vi "CreateLib.vi"(0 "LibWriter":refnum<class "LibWriter.lvclass">, 1 "ProjectTreePosition(String or Project Item Ref)":variant, 2 "CreateLibData":T1, 5 "error in (no error)":errorcluster, 6 "KeepLvLibRefOpen(False)":bool, 7 "HeaderToApply (take from VIRef or /use 2D-8bit header, Ignored if not wired)":variant) -> (14 "LibWriter":refnum<class "LibWriter.lvclass">, 15 "LVLibLibraryRefnum":refnum<vi>, 16 "TemplateVersionUsed":string, 19 "error out":errorcluster)   [LabVIEW 2014, in "LibWriter.lvclass"]
uses:
  <resource>/Framework/Providers/Open_GDS/ClassProviders/LibProvider_BaseClassInterface/LibWriter_class/ClassWriter_class/LibWriter.lvclass
  <resource>/Framework/Providers/Open_GDS/ClassProviders/LibProvider_BaseClassInterface/LibWriter_class/CreateLibData.vi
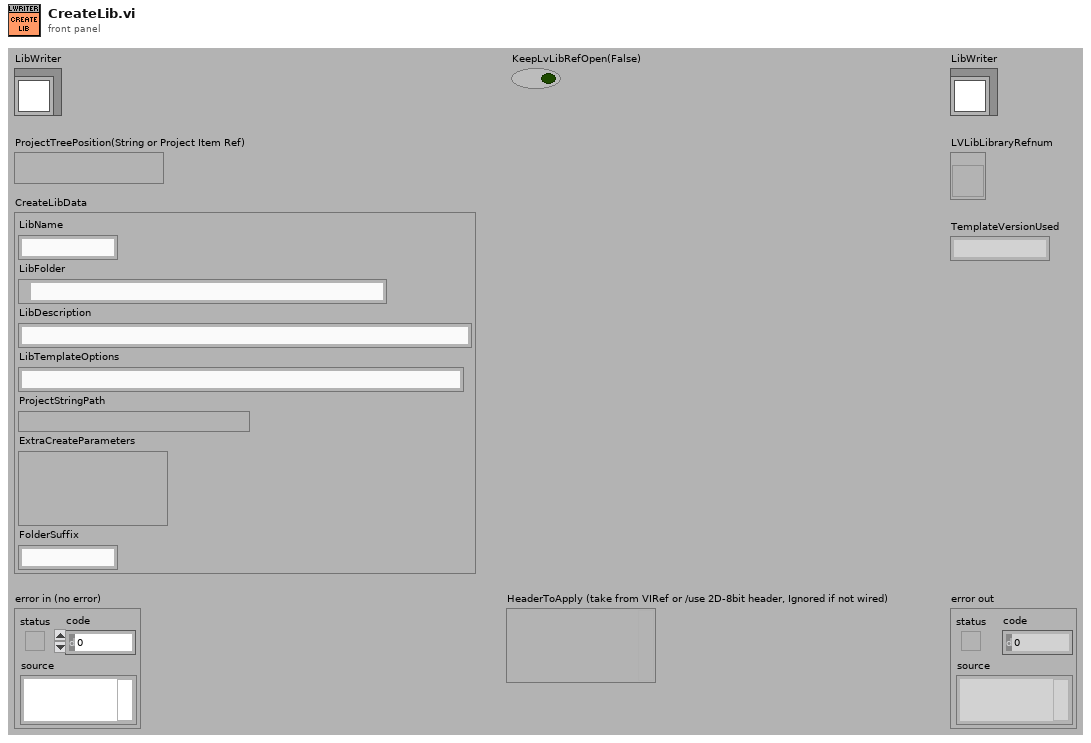
[diagram p1: front panel]
types:
  T1 = typedef "LibWriter.lvclass/CreateLibData.vi" = cluster{"LibName":string, "LibFolder":path, "LibDescription":string, "LibTemplateOptions":string, "ProjectStringPath":variant, "ExtraCreateParameters":variant, "FolderSuffix":string}
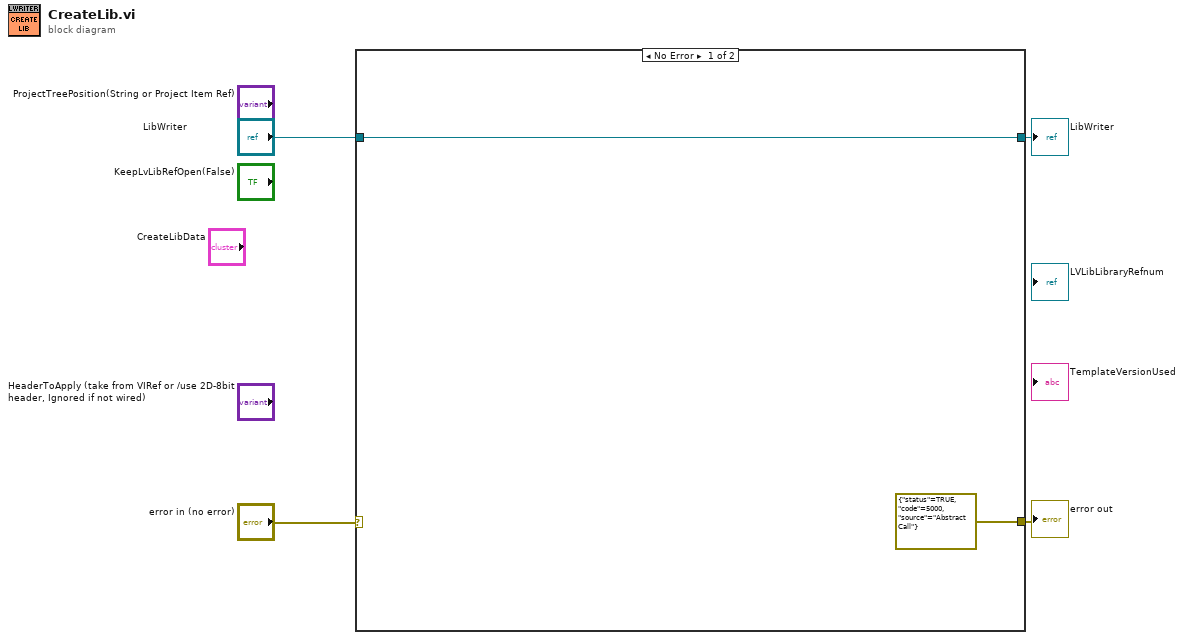
[diagram p0: block diagram]
diagram:
  n1 = case shown="No Error" "error in (no error)" {
    selector: "error in (no error)" -> [_ w7]
    tunnel: "LibWriter" -> [w5 w8]
    tunnel: [errorcluster {"status"=TRUE, "code"=5000, "source"="Abstract Call"} ("error IO") w7] -> w3
    tunnel: [w5 w8] -> w2
    frame No Error {
    }
    frame Error {
    }
  }
  "LibWriter" <- w2
  "error out" <- w3
